vi "Actor Core.vi"(8 "error in":errorcluster, 11 "TestProcesses.lvlib:Counter.lvclass":refnum<class "Counter.lvclass">) -> (0 "error out":errorcluster, 3 "Actor out":refnum<class "Actor.lvclass">)   [LabVIEW 2020, in "TestProcesses.lvlib" / "Counter.lvclass"]
doc: "(<B>Filename</B>: Actor Framework.lvlib:Actor.lvclass:Actor Core.vi)\n\nReceives messages to the actor, reacts to them, and initiates any error handling that may shut the actor down.\n\nDescendant classes may override this VI to append parallel tasks for the actor to complete while it handles messages. Overrides use the Call Parent Class Method node."
uses:
  Counter.lvclass
  <vilib>/ActorFramework/Actor/Actor.lvclass
  C:/Program Files (x86)/National Instruments/LabVIEW 2020/vi.lib/ActorFramework/Actor/Actor.lvclass
  Counter.lvclass/Counter.ctl
  <vilib>/ActorFramework/Actor/Actor.lvclass/Actor.ctl
  <vilib>/ActorFramework/Message Enqueuer/Message Enqueuer.lvclass/Message Enqueuer.ctl
  <vilib>/ActorFramework/Message Enqueuer/Init from Existing Queue.vi
  <vilib>/ActorFramework/Message Enqueuer/Enqueue.vi
  <vilib>/ActorFramework/Stop Msg/Stop Msg.lvclass
  C:/Program Files (x86)/National Instruments/LabVIEW 2020/vi.lib/ActorFramework/Message/Message.lvclass
  <vilib>/ActorFramework/Message Priority Queue/Priority Enqueue.vi
  <vilib>/ActorFramework/Message Enqueuer/Message Enqueuer.lvclass
  ServiceManager/ServiceManager/DownstreamMsg/DownStreamMsgHandler.lvclass
  C:/Users/taylo/Projects/g-go-service-fwrk/scratchpad/ServiceManagerBeta/ServiceManager/ServiceManager/DownstreamMsg/DownStreamMsgHandler.lvclass
  C:/Users/taylo/Projects/g-go-service-fwrk/scratchpad/ServiceManagerBeta/Test/Processes/Counter/Counter.lvclass
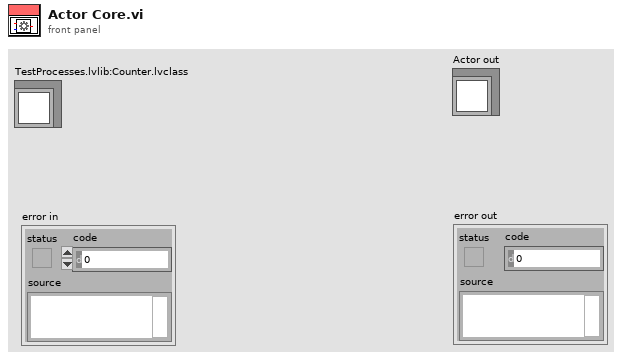
[diagram p1: front panel]
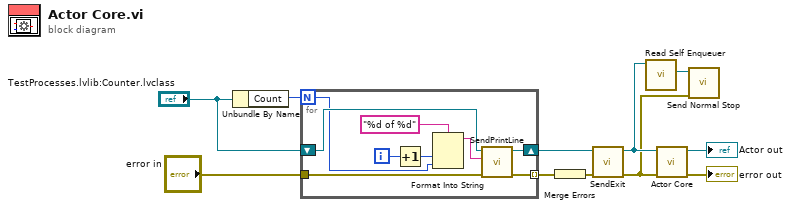
[diagram p0: block diagram]
diagram:
  n1 = Unbundle By Name("TestProcesses.lvlib:Counter.lvclass") -> ("Count"=w9:u32)
  n2 = for {
    N: w9 -> [w16]
    shift-right: [w19] -> w4
    shift-left: "TestProcesses.lvlib:Counter.lvclass" -> [w20]
    tunnel: "error in" -> [w13]
    tunnel: [w12] -> w7 mode=indexing
    i -> [w18]
    n3 = Increment(x=w18) -> (x+1=w14:i32)
    n4 = Format Into String(format string="%d of %d", w14, w16) -> (resulting string=w17:string)  [unwired: 2 in, 1 out]
    n5 = call-dynamic "SendPrintLine.vi"("error in (no error)"=w13, "e"=w17, "DownStreamMsgHandler in"=w20) -> ("error out"=w12:errorcluster, "DownStreamMsgHandler out"=w19:refnum<class "Counter.lvclass">)  [unwired: 7 in]
  }
  n6 = Merge Errors(w7) -> (w5:errorcluster)
  n7 = call-dynamic "SendExit.vi"("error in (no error)"=w5, "DownStreamMsgHandler in"=w4) -> ("error out"=w2:errorcluster, "DownStreamMsgHandler out"=w3:refnum<class "Counter.lvclass">)  [unwired: 8 in]
  n8 = call <vilib>:"Read Self Enqueuer.vi"("Actor"=w3) -> ("Self Enqueuer"=w6:refnum<class "Message Enqueuer.lvclass">)  [unwired: 10 in]
  n9 = call-parent "Actor Core.vi"("error in"=w2, "Actor in"=w3) -> ("error out"=→"error out":errorcluster, "Actor out"=→"Actor out":refnum<class "Actor.lvclass">)  [unwired: 8 in]
  n10 = call <vilib>:"Send Normal Stop.vi"("error in (no error)"=w2, "Message Enqueuer"=w6) -> ()  [unwired: 9 in, 1 out]
